vi "getAdditionalDataFromXML.vi"(8 "error in (no error)":errorcluster, 10 "Xml":refnum<class "xmlNode.lvclass">, 11 "RampEvent in":refnum<class "RampEvent.lvclass">) -> (0 "error out":errorcluster, 2 "Xml out":refnum<class "xmlNode.lvclass">, 3 "RampEvent out":refnum<class "RampEvent.lvclass">)   [LabVIEW 2009, in "Tools.lvlib" / "Scripting.lvlib" / "RampEvent.lvclass"]
uses:
  RampEvent.lvclass
  xmlNode/xmlNode.lvclass
  RampEvent.lvclass/RampEvent.ctl
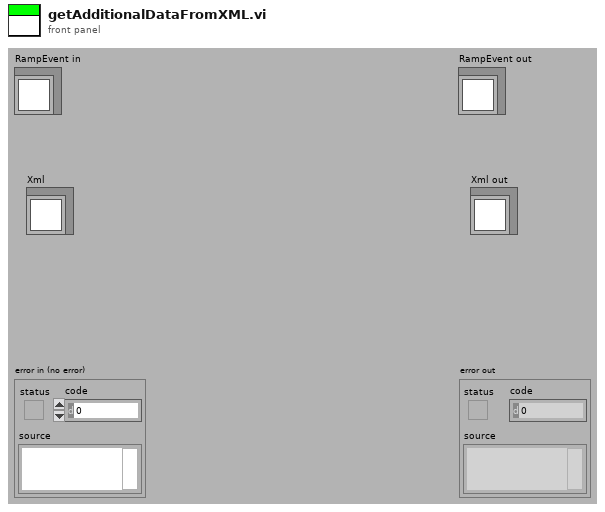
[diagram p1: front panel]
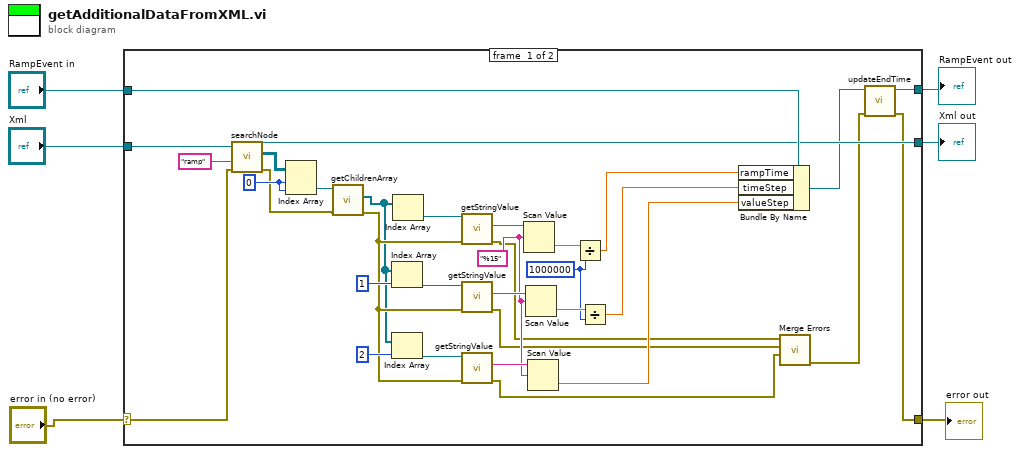
[diagram p0: block diagram]
diagram:
  n1 = case shown="No Error" "error in (no error)" {
    selector: "error in (no error)" -> [w31 w40]
    tunnel: [w7 w40] -> w5
    tunnel: "RampEvent in" -> [w18 w42]
    tunnel: [w9 w42] -> w3
    tunnel: "Xml" -> [w32 w41]
    tunnel: [w17 w41] -> w1
    frame #0 {
      w21 = 1000000
      w15 = "%15"
      w37 = 0
      n2 = call-dynamic "searchNode.vi"("error in (no error)"=w31, "searchElementName"="ramp", "xmlNode in"=w32) -> ("error out"=w35:errorcluster, "arrayXmlNodes"=w38:refnum<class "xmlNode.lvclass">[][], "xmlNode out"=w17:refnum<class "xmlNode.lvclass">)  [unwired: 6 in]
      n3 = Index Array(array=w38, index (row)=w37, index (col)=w37) -> (element=w36:refnum<class "xmlNode.lvclass">)
      n4 = call-dynamic "getChildrenArray.vi"("error in (no error)"=w35, "xmlNode.lvclass in"=w36) -> ("error out"=w27:errorcluster, "Children"=w26:refnum<class "xmlNode.lvclass">[])  [unwired: 7 in, 1 out]
      n5 = Index Array(array=w26, index=1) -> (element=w33:refnum<class "xmlNode.lvclass">)
      n6 = Index Array(array=w26, index=2) -> (element=w29:refnum<class "xmlNode.lvclass">)
      n7 = Index Array(array=w26) -> (element=w34:refnum<class "xmlNode.lvclass">)  [unwired: 1 in]
      n8 = call-dynamic "getStringValue.vi"("error in (no error)"=w27, "xmlNode.lvclass in"=w34) -> ("error out"=w13:errorcluster, "stringValue"=w25:string)  [unwired: 7 in, 1 out]
      n9 = call-dynamic "getStringValue.vi"("error in (no error)"=w27, "xmlNode.lvclass in"=w33) -> ("error out"=w12:errorcluster, "stringValue"=w24:string)  [unwired: 7 in, 1 out]
      n10 = call-dynamic "getStringValue.vi"("error in (no error)"=w27, "xmlNode.lvclass in"=w29) -> ("error out"=w11:errorcluster, "stringValue"=w16:string)  [unwired: 7 in, 1 out]
      n11 = Scan Value(string=w25, format string=w15) -> (value=w23:dbl)  [unwired: 1 in, 1 out]
      n12 = Scan Value(string=w24, format string=w15) -> (value=w22:dbl)  [unwired: 1 in, 1 out]
      n13 = Scan Value(string=w16, format string=w15) -> (value=w14:dbl)  [unwired: 1 in, 1 out]
      n14 = Divide(x=w23, y=w21) -> (x/y=w20:dbl)
      n15 = Divide(x=w22, y=w21) -> (x/y=w19:dbl)
      n16 = Bundle By Name(cluster=w18, "rampTime"=w20, "timeStep"=w19, "valueStep"=w14) -> (w10:refnum<class "RampEvent.lvclass">)
      n17 = call <vilib>:"Merge Errors.vi"("error in 3 (no error)"=w11, "error in 2 (no error)"=w12, "error in 1 (no error)"=w13) -> ("error out"=w8:errorcluster)  [unwired: 4 in]
      n18 = call-dynamic "updateEndTime.vi"("error in (no error)"=w8, "RampEvent in"=w10) -> ("error out"=w7:errorcluster, "RampEvent out"=w9:refnum<class "RampEvent.lvclass">)  [unwired: 8 in]
    }
    frame #1 {
    }
  }
  "error out" <- w5
  "RampEvent out" <- w3
  "Xml out" <- w1
